vi "Angle Mesurement.vi"() -> ()   [LabVIEW 2016]
uses:
  <vilib>/vision/Measure.llb/Edge Options.ctl
  <vilib>/vision/Measure.llb/Edge Polarity.ctl
  <vilib>/vision/NI_Vision_Development_Module.lvlib
panel:
  out "Angle (Pixel) 3":dbl format="%#_4g"
  out "Angle (Pixel) 2":dbl format="%#_4g"
  out "Angle (Pixel)":dbl format="%#_4g"
  out "Fitted Line":T1 {"Straightness" format="%.2f"; "Angle (Real World)" format="%.2f"; "Line Segment (Real World)"."Point 2"."Y" format="%.2f"; "Line Segment (Real World)"."Point 2"."X" format="%.2f"; "Line Segment (Real World)"."Point 1"."Y" format="%.2f"; "Line Segment (Real World)"."Point 1"."X" format="%.2f"; "Average SNR (dB)" format="%.2f"; "Average Strength" format="%.2f"; "Angle (Pixel)" format="%.2f"; "Line Segment (Pixels)"."Point 2"."Y" format="%.2f"; "Line Segment (Pixels)"."Point 2"."X" format="%.2f"; "Line Segment (Pixels)"."Point 1"."Y" format="%.2f"; "Line Segment (Pixels)"."Point 1"."X" format="%.2f"}
  in  "Options3":T4={"Scan Direction"=0, "Edge Options"={"Edge Polarity"=2, "Kernel Size"=3, "Width"=3, "Minimum Edge Strength"=10.0, "Interpolation Type"=enum."Bilinear Fixed", "Data Processing Method"=enum."Average"}, "Show Search Area"=TRUE, "Show Search Lines"=TRUE, "Show Edges Found"=TRUE, "Show Result"=TRUE, "Search Area Color"=65280, "Search Lines Color"=255, "Edge Locations Color"=16776960, "Result Color"=16711680, "Overlay Group Name"=""} {"Scan Direction" items=["Counter-Clockwise", "Clockwise"]; "Edge Options"."Edge Polarity" items=["All Edges", "Rising Edges", "Falling Edges"]; "Edge Options"."Minimum Edge Strength" format="%.2f"; "Edge Options"."Width" step=2; "Edge Options"."Kernel Size" step=2}
  in  "Annulus":T5={"Center X"=40, "Center Y"=220, "Inner Radius"=40, "Outer Radius"=80, "Start Angle"=0.0, "End Angle"=180.0} {"End Angle" min=-90.0 max=90.0 step=1.0 format="%.2f"; "Start Angle" min=-90.0 max=90.0 step=1.0 format="%.2f"; "Center X" scale=0.0..1024.0}
  out "Straight Edges 2":T6(array[cluster]) {"Point2 (Real-World)"."Y" format="%.2f"; "Point2 (Real-World)"."X" format="%.2f"; "Point1 (Real-World)"."Y" format="%.2f"; "Point1 (Real-World)"."X" format="%.2f"; "Point2 (Pixels)"."Y" format="%.2f"; "Point2 (Pixels)"."X" format="%.2f"; "Point1 (Pixels)"."Y" format="%.2f"; "Point1 (Pixels)"."X" format="%.2f"}
  out "Straight Edges":T6(array[cluster]) {"Point2 (Real-World)"."Y" format="%.2f"; "Point2 (Real-World)"."X" format="%.2f"; "Point1 (Real-World)"."Y" format="%.2f"; "Point1 (Real-World)"."X" format="%.2f"; "Point2 (Pixels)"."Y" format="%.2f"; "Point2 (Pixels)"."X" format="%.2f"; "Point1 (Pixels)"."Y" format="%.2f"; "Point1 (Pixels)"."X" format="%.2f"}
  in  "Options2":T7={"Search Direction"=3, "Edge Options"={"Edge Polarity"=0, "Kernel Size"=3, "Width"=3, "Minimum Edge Strength"=10.0, "Interpolation Type"=enum."Bilinear Fixed", "Data Processing Method"=enum."Average"}, "Show Search Area"=TRUE, "Show Search Lines"=TRUE, "Show Edges Found"=TRUE, "Show Result"=TRUE, "Search Area Color"=65280, "Search Lines Color"=255, "Edge Locations Color"=16776960, "Result Color"=16711680, "Overlay Group Name"=""} {"Edge Options"."Edge Polarity" items=["All Edges", "Rising Edges", "Falling Edges"]; "Edge Options"."Minimum Edge Strength" format="%.2f"; "Edge Options"."Width" step=2; "Edge Options"."Kernel Size" step=2; "Search Direction" items=["Left to Right", "Right to Left", "Top to Bottom", "Bottom to Top"]}
  in  "Options":T7={"Search Direction"=0, "Edge Options"={"Edge Polarity"=0, "Kernel Size"=3, "Width"=3, "Minimum Edge Strength"=10.0, "Interpolation Type"=enum."Bilinear Fixed", "Data Processing Method"=enum."Average"}, "Show Search Area"=TRUE, "Show Search Lines"=TRUE, "Show Edges Found"=TRUE, "Show Result"=TRUE, "Search Area Color"=65280, "Search Lines Color"=255, "Edge Locations Color"=16776960, "Result Color"=16711680, "Overlay Group Name"=""} {"Edge Options"."Edge Polarity" items=["All Edges", "Rising Edges", "Falling Edges"]; "Edge Options"."Minimum Edge Strength" format="%.2f"; "Edge Options"."Width" step=2; "Edge Options"."Kernel Size" step=2; "Search Direction" items=["Left to Right", "Right to Left", "Top to Bottom", "Bottom to Top"]}
  in  "Rectangle2":T8={"Left"=167, "Top"=134, "Right"=240, "Bottom"=218, "Rotation"=0.0} {"Rotation" min=-90.0 max=90.0 step=1.0 format="%.2f"; "Left" scale=0.0..1024.0; "Right" scale=0.0..1024.0}
  in  "Rectangle":T8={"Left"=50, "Top"=106, "Right"=150, "Bottom"=140, "Rotation"=0.0} {"Rotation" min=-90.0 max=90.0 step=1.0 format="%.2f"; "Left" scale=0.0..1024.0; "Right" scale=0.0..1024.0}
  out "Image":T9(plugin-control)
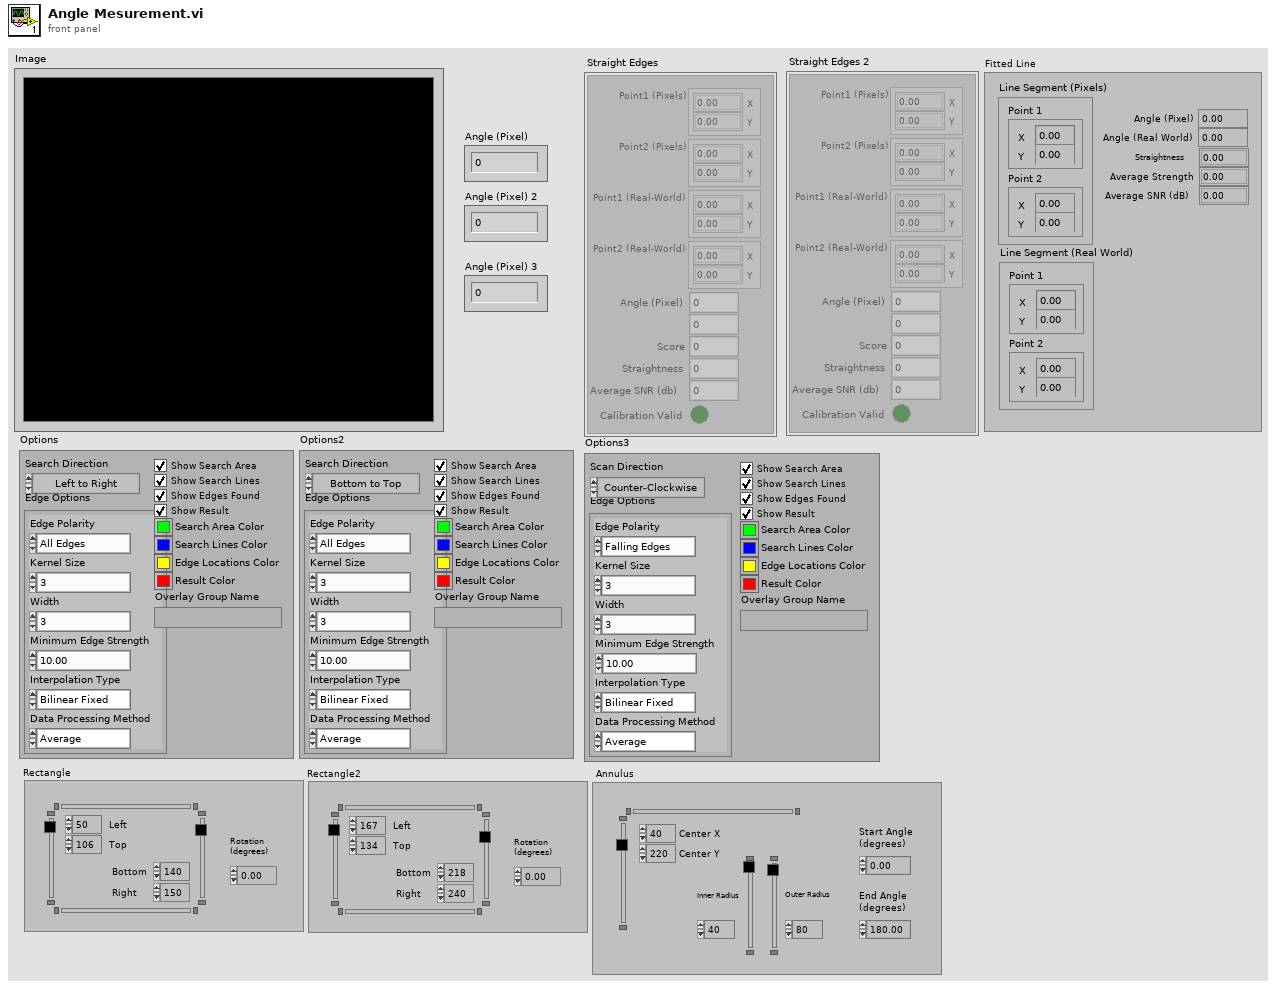
[diagram p1: front panel]
types:
  T1 = cluster{"Line Segment (Pixels)":cluster{"Point 1":cluster{"X":sgl, "Y":sgl}, "Point 2":cluster{"X":sgl, "Y":sgl}}, "Line Segment (Real World)":cluster{"Point 1":cluster{"X":sgl, "Y":sgl}, "Point 2":cluster{"X":sgl, "Y":sgl}}, "Angle (Pixel)":dbl, "Angle (Real World)":dbl, "Straightness":dbl, "Average Strength":dbl, "Average SNR (dB)":dbl}
  T2 = typedef "Edge Options.ctl" = cluster{"Edge Polarity":T3, "Kernel Size":u32, "Width":u32, "Minimum Edge Strength":sgl, "Interpolation Type":enum32{"Zero Order", "Bilinear", "Quadratic", "Cubic", "Bilinear Fixed"}, "Data Processing Method":enum32{"Average", "Median"}}
  T3 = typedef "Edge Polarity.ctl" = u32
  T4 = cluster{"Scan Direction":u16, "Edge Options":T2, "Show Search Area":bool, "Show Search Lines":bool, "Show Edges Found":bool, "Show Result":bool, "Search Area Color":u32, "Search Lines Color":u32, "Edge Locations Color":u32, "Result Color":u32, "Overlay Group Name":string}
  T5 = typedef "IMAQ Circle" = cluster{"Center X":i32, "Center Y":i32, "Inner Radius":i32, "Outer Radius":i32, "Start Angle":dbl, "End Angle":dbl}
  T6 = cluster{"Point1 (Pixels)":cluster{"X":sgl, "Y":sgl}, "Point2 (Pixels)":cluster{"X":sgl, "Y":sgl}, "Point1 (Real-World)":cluster{"X":sgl, "Y":sgl}, "Point2 (Real-World)":cluster{"X":sgl, "Y":sgl}, "Angle (Pixel)":dbl, "Angle (Real-World)":dbl, "Score":dbl, "Straightness":dbl, "Average SNR (db)":dbl, "Calibration Valid":bool}[]
  T7 = cluster{"Search Direction":u32, "Edge Options":T2, "Show Search Area":bool, "Show Search Lines":bool, "Show Edges Found":bool, "Show Result":bool, "Search Area Color":u32, "Search Lines Color":u32, "Edge Locations Color":u32, "Result Color":u32, "Overlay Group Name":string}
  T8 = typedef "IMAQ Rectangle" = cluster{"Left":i32, "Top":i32, "Right":i32, "Bottom":i32, "Rotation":dbl}
  T9 = typedef "IMAQ Image.ctl" = refnum<image>
  T10 = typedef "ROI Descriptor" = cluster{"Global Rectangle":i32[], "Contours":cluster{"ID":enum32{"External", "Internal"}, "Type":u32, "Coordinates":i32[]}[]}
  T11 = cluster{"Point1 (Pixels)":cluster{"X":sgl, "Y":sgl}, "Point2 (Pixels)":cluster{"X":sgl, "Y":sgl}, "Point1 (Real-World)":cluster{"X":sgl, "Y":sgl}, "Point2 (Real-World)":cluster{"X":sgl, "Y":sgl}, "Angle (Pixel)":dbl, "Angle (Real-World)":dbl, "Score":dbl, "Straightness":dbl, "Average SNR (db)":dbl, "Calibration Valid":bool}
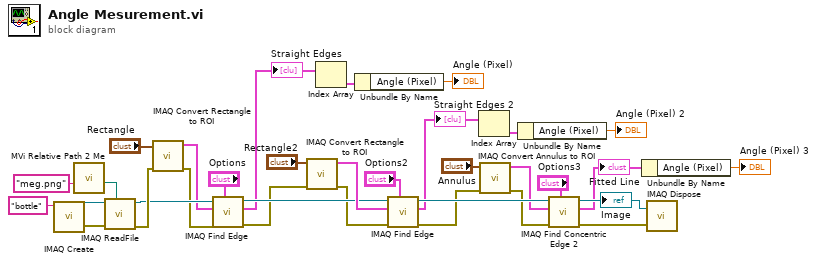
[diagram p0: block diagram]
diagram:
  n1 = call "IMAQ Create"("Image Name"="bottle") -> ("Src"=w31:T9, "error out"=w32:errorcluster)  [unwired: 4 in]
  n2 = call "MVi Relative Path 2 Me.vi"("Relative Path"="meg.png" ("Image Name")) -> ("Appended Dir"=w30:path)  [unwired: 5 in, 1 out]
  n3 = call "IMAQ ReadFile"("File Path"=w30, "error in (no error)"=w32, "Image"=w31) -> ("error out"=w29:errorcluster, "Image Out"=w27:T9)  [unwired: 4 in, 3 out]
  n4 = call "IMAQ Convert Rectangle to ROI"("error in (no error)"=w29, "Rectangle"="Rectangle") -> ("error out"=w19:errorcluster, "ROI Descriptor"=w26:T10)  [unwired: 7 in]
  n5 = call "IMAQ Find Edge"("Options"="Options", "error in (no error)"=w19, "ROI Descriptor"=w26, "Image"=w27) -> ("error out"=w18:errorcluster, "Straight Edges"=w8:T6, "Image Out"=w24:T9)  [unwired: 4 in, 1 out]
  "Straight Edges" <- w8
  n6 = call "IMAQ Convert Rectangle to ROI"("error in (no error)"=w18, "Rectangle"="Rectangle2") -> ("error out"=w17:errorcluster, "ROI Descriptor"=w25:T10)  [unwired: 7 in]
  n7 = Index Array(array=w8) -> (element=w7:T11)  [unwired: 1 in]
  n8 = Unbundle By Name(w7) -> ("Angle (Pixel)"=→"Angle (Pixel)":dbl)
  n9 = call "IMAQ Find Edge"("Options"="Options2", "error in (no error)"=w17, "ROI Descriptor"=w25, "Image"=w24) -> ("error out"=w14:errorcluster, "Straight Edges"=w4:T6, "Image Out"=w16:T9)  [unwired: 4 in, 1 out]
  "Straight Edges 2" <- w4
  n10 = Index Array(array=w4) -> (element=w5:T11)  [unwired: 1 in]
  n11 = call "IMAQ Convert Annulus to ROI"("error in (no error)"=w14, "Annulus"="Annulus") -> ("error out"=w13:errorcluster, "ROI Descriptor"=w12:T10)  [unwired: 7 in]
  n12 = Unbundle By Name(w5) -> ("Angle (Pixel)"=→"Angle (Pixel) 2":dbl)
  n13 = call "IMAQ Find Concentric Edge 2"("Options"="Options3", "error in (no error)"=w13, "ROI Descriptor"=w12, "Image"=w16) -> ("error out"=w11:errorcluster, "Fitted Line"=w1:T1, "Image Out"=w10:T9)  [unwired: 3 in, 2 out]
  "Image" <- w10
  "Fitted Line" <- w1
  n14 = Unbundle By Name(w1) -> ("Angle (Pixel)"=→"Angle (Pixel) 3":dbl)
  n15 = call "IMAQ Dispose"("Image"=w10, "error in (no error)"=w11) -> ()  [unwired: 4 in, 1 out]
